vi "HaberlesmeKart.vi"(0 "error in (no error)":errorcluster, 2 "VISA resource name":refnum<visa-resource-name>="COM1", 3 "Voltaj set":dbl) -> (4 "error out":errorcluster, 5 "Voltaj":dbl, 8 "Akım":dbl)   [LabVIEW 2016]
panel:
  out "c string":string
  out "s3":string
  out "s2":string
  out "s1":string
  out "read string":string
  out "string 4":string
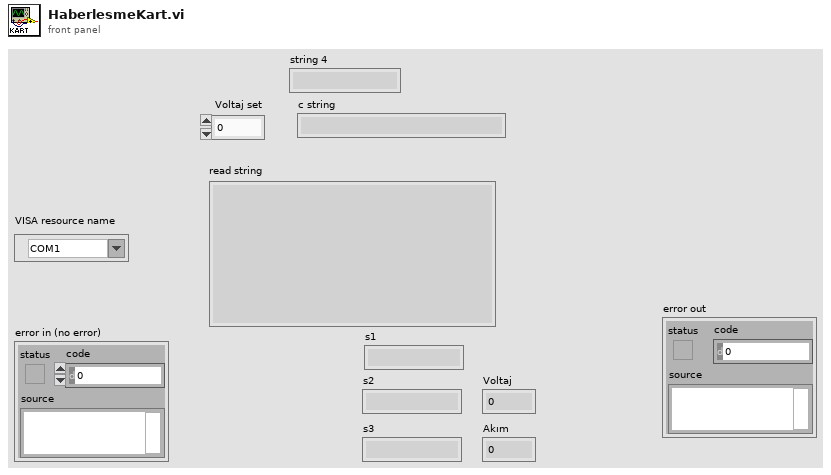
[diagram p1: front panel]
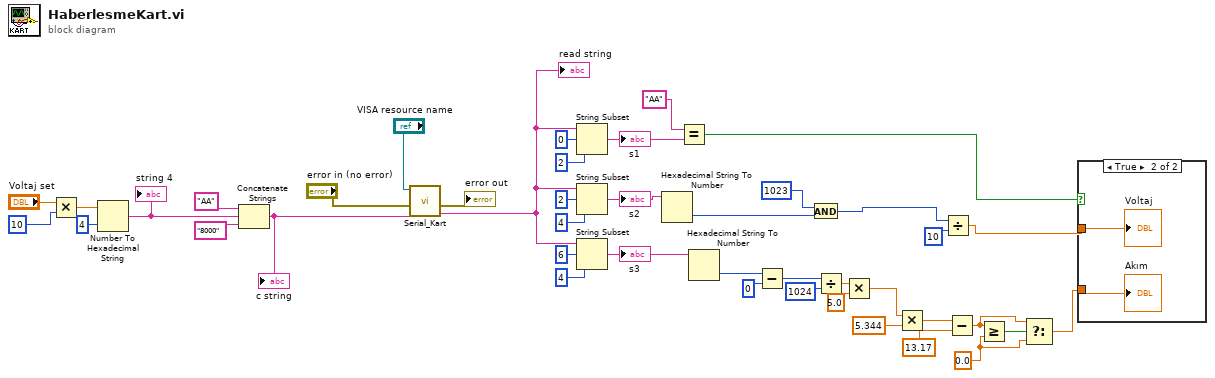
[diagram p0: block diagram]
diagram:
  w5 = 0.0 ("y")
  n1 = Multiply(x="Voltaj set", y=u16 10) -> (x*y=w25:dbl)
  n2 = Number To Hexadecimal String(1:i16 4 ("width (-)"), 2:w25) -> (0:w21:string)
  "string 4" <- w21
  n3 = Concatenate Strings("AA" ("element"), w21, "8000" ("string")) -> (w42:string)
  "c string" <- w42
  n4 = call "Serial_Kart.vi"("string to write"=w42, "error in (no error)"="error in (no error)", "VISA resource name"="VISA resource name") -> ("read string"=w33:string, "error out"=→"error out":errorcluster)  [unwired: 3 in]
  "read string" <- w33
  n5 = String Subset(string=w33, offset (0)=0, length (rest)=2 ("length (rest)")) -> (substring=w30:string)
  "s1" <- w30
  n6 = String Subset(string=w33, offset (0)=2, length (rest)=4 ("length (rest)")) -> (substring=w32:string)
  "s2" <- w32
  n7 = String Subset(string=w33, offset (0)=6, length (rest)=4 ("length (rest)")) -> (substring=w31:string)
  "s3" <- w31
  n8 = Hexadecimal String To Number(string=w32) -> (number=w24:u32)  [unwired: 2 in, 1 out]
  n9 = Equal?(x="AA", y=w30) -> (x = y?=w28:bool)
  n10 = Hexadecimal String To Number(string=w31) -> (number=w17:u32)  [unwired: 2 in, 1 out]
  n11 = Subtract(x=w17, y=u32 0) -> (x-y=w16:u32)
  n12 = And(x=u32 1023, y=w24) -> (x .and. y?=w3:u32)
  n13 = Divide(x=w16, y=u32 1024) -> (x/y=w19:dbl)
  n14 = Multiply(x=w19, y=5.0) -> (x*y=w11:dbl)
  n15 = Multiply(x=w11, y=5.344) -> (x*y=w9:dbl)
  n16 = Divide(x=w3, y=u16 10) -> (x/y=w1:dbl)
  n17 = Subtract(x=w9, y=13.17) -> (x-y=w6:dbl)
  n18 = Greater Or Equal?(x=w6, y=w5) -> (x >= y?=w7:bool)
  n19 = Select(t=w6, s=w7, f=w5) -> (s? t:f=w4:dbl)
  n20 = case shown="True" w28 {
    tunnel: w1 -> [_ w44]
    tunnel: w4 -> [_ w43]
    frame False {
    }
    frame True {
      "Voltaj" <- w44
      "Akım" <- w43
    }
  }
